vi "CloseIO.vi"   [LabVIEW 2012]
uses:
  <vilib>/Rock Robotics/WPI/RobotDrive/WPI_RobotDriveGetSetRefNum.vi
types:
  T1 = typedef "WPI_UltrasonicDeviceRef.ctl" = cluster{"DevStatus":errorcluster, "Ping Digital Module":T2, "Echo Digital Module":T2, "Ping Channel":T3, "Echo Channel":T3, "CntIndex":T4}
  T2 = typedef "FPGA_TypedefDigitalModule.ctl" = enum16{"Digital Module 1", "Digital Module 2"}
  T3 = typedef "FPGA_DIOChannel.ctl" = enum8{"DIO 1", "DIO 2", "DIO 3", "DIO 4", "DIO 5", "DIO 6", "DIO 7", "DIO 8", "DIO 9", "DIO 10", "DIO 11", "DIO 12", "DIO 13", "DIO 14", "Invalid"}
  T4 = typedef "FPGA_CounterCtrSystemIndex.ctl" = enum8{"Ctr 0", "Ctr 1", "Ctr 2", "Ctr 3", "Ctr 4", "Ctr 5", "Ctr 6", "Ctr 7", "Invalid"}
  T5 = typedef "WPI_MotorControlDeviceRef.ctl" = cluster{"DeviceStatus":errorcluster, "Type":enum16{"PWM", "CAN"}, "PWM":cluster{"Digital Module":T2, "PWM Channel":T6, "DeadBand":T7}, "CAN":cluster{"Device Number":u8, "Control Mode":T8, "Semaphore":T9, "Max Vout":dbl}, "Invert":bool, "TransformRef":T10, "InvTransformRef":T10}
  T6 = typedef "FPGA_DIOPWMChannel.ctl" = enum8{"PWM 1", "PWM 2", "PWM 3", "PWM 4", "PWM 5", "PWM 6", "PWM 7", "PWM 8", "PWM 9", "PWM 10", "Invalid"}
  T7 = typedef "WPI_PWMDeadband.ctl" = cluster{"Name":string, "maxPositivePwm":i32, "minPositivePwm":i32, "centerPwm":i32, "maxNegativePwm":i32, "minNegativePwm":i32, "angularRange":u16}
  T8 = typedef "WPI_CANJaguar_ControlMode.ctl" = enum8{"Percent VBus", "Current", "Speed", "Position", "Voltage"}
  T9 = typedef "Semaphore RefNum" = refnum<k1>
  T10 = typedef "WPI_PWMTransform_ConPane.ctl" = refnum<vi>
  T11 = typedef "WPI_RobotDriveDevRef.ctl" = cluster{"DevStatus":errorcluster, "Motors[]":T5[], "Square Inputs":bool, "Max Output":dbl, "Isochronous":bool}
  T12 = typedef "WPI_DigitalInputDevRef.ctl" = cluster{"DevStatus":errorcluster, "DIO Channel":T3, "Digital Module":T2}
  T13 = typedef "WPI_CounterDevRef.ctl" = cluster{"DevStatus":errorcluster, "CntIndex":T4}
  T14 = typedef "WPI_EncoderDevRef.ctl" = cluster{"DevStatus":errorcluster, "EncoderIndex":T15, "CounterIndex":T4, "DistancePerCount":dbl, "Decoding Type":T16}
  T15 = typedef "FPGA_EncoderIdx.ctl" = enum8{"Enc 0", "Enc 1", "Enc 2", "Enc 3", "Invalid"}
  T16 = typedef "WPI_EncoderType.ctl" = enum16{"1x", "2x", "4x"}
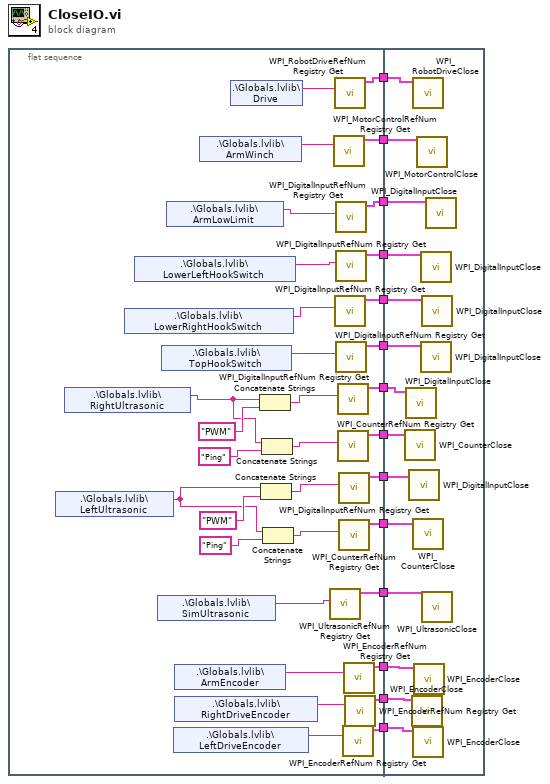
[diagram p0: block diagram]
diagram:
  n1 = flat-sequence {
    tunnel: [w46] -> w14
    tunnel: [w45] -> w13
    tunnel: [w30] -> w12
    tunnel: [w29] -> w11
    tunnel: [w28] -> w10
    tunnel: [w27] -> w9
    tunnel: [w26] -> w8
    tunnel: [w25] -> w7
    tunnel: [w24] -> w6
    tunnel: [w23] -> w5
    tunnel: [w21] -> w4
    tunnel: [w20] -> w3
    tunnel: [w17] -> w2
    tunnel: [w15] -> w1
    tunnel: w14 -> [w62]
    tunnel: w13 -> [w61]
    tunnel: w12 -> [w60]
    tunnel: w11 -> [w59]
    tunnel: w10 -> [w58]
    tunnel: w9 -> [w57]
    tunnel: w8 -> [w56]
    tunnel: w7 -> [w55]
    tunnel: w6 -> [w54]
    tunnel: w5 -> [w53]
    tunnel: w4 -> [w52]
    tunnel: w3 -> [w51]
    tunnel: w2 -> [w50]
    tunnel: w1 -> [w49]
    frame #0 {
      n2 = shared-variable ".\\Globals.lvlib\\LeftUltrasonic"() -> (w32:string)  [unwired: 1 in, 1 out]
      n3 = shared-variable ".\\Globals.lvlib\\RightUltrasonic"() -> (w38:string)  [unwired: 1 in, 1 out]
      n4 = shared-variable ".\\Globals.lvlib\\LowerRightHookSwitch"() -> (w42:string)  [unwired: 1 in, 1 out]
      n5 = shared-variable ".\\Globals.lvlib\\LowerLeftHookSwitch"() -> (w43:string)  [unwired: 1 in, 1 out]
      n6 = shared-variable ".\\Globals.lvlib\\SimUltrasonic"() -> (w16:string)  [unwired: 1 in, 1 out]
      n7 = shared-variable ".\\Globals.lvlib\\TopHookSwitch"() -> (w41:string)  [unwired: 1 in, 1 out]
      n8 = shared-variable ".\\Globals.lvlib\\ArmLowLimit"() -> (w44:string)  [unwired: 1 in, 1 out]
      n9 = shared-variable ".\\Globals.lvlib\\LeftDriveEncoder"() -> (w18:string)  [unwired: 1 in, 1 out]
      n10 = shared-variable ".\\Globals.lvlib\\ArmEncoder"() -> (w19:string)  [unwired: 1 in, 1 out]
      n11 = shared-variable ".\\Globals.lvlib\\RightDriveEncoder"() -> (w22:string)  [unwired: 1 in, 1 out]
      n12 = shared-variable ".\\Globals.lvlib\\ArmWinch"() -> (w47:string)  [unwired: 1 in, 1 out]
      n13 = shared-variable ".\\Globals.lvlib\\Drive"() -> (w48:string)  [unwired: 1 in, 1 out]
      n14 = Concatenate Strings(w38, "PWM") -> (w39:string)
      n15 = Concatenate Strings(w32, "PWM") -> (w34:string)
      n16 = Concatenate Strings(w38, "Ping") -> (w36:string)
      n17 = Concatenate Strings(w32, "Ping") -> (w35:string)
      n18 = call <vilib>:"WPI_UltrasonicRefNum Registry Get.vi"("refnum name"=w16) -> ("UltrasonicDevRef"=w15:T1)  [unwired: 9 in, 1 out]
      n19 = call <vilib>:"WPI_MotorControlRefNum Registry Get.vi"("refnum name"=w47) -> ("MotorControlDevRef"=w45:T5)  [unwired: 9 in, 1 out]
      n20 = call <vilib>:"WPI_RobotDriveRefNum Registry Get.vi"("refnum name"=w48) -> ("RobotDriveDevRef"=w46:T11)  [unwired: 9 in, 1 out]
      n21 = call <vilib>:"WPI_DigitalInputRefNum Registry Get.vi"("refnum name"=w42) -> ("DigitalInputDevRef"=w27:T12)  [unwired: 9 in, 1 out]
      n22 = call <vilib>:"WPI_DigitalInputRefNum Registry Get.vi"("refnum name"=w44) -> ("DigitalInputDevRef"=w25:T12)  [unwired: 9 in, 1 out]
      n23 = call <vilib>:"WPI_DigitalInputRefNum Registry Get.vi"("refnum name"=w43) -> ("DigitalInputDevRef"=w26:T12)  [unwired: 9 in, 1 out]
      n24 = call <vilib>:"WPI_DigitalInputRefNum Registry Get.vi"("refnum name"=w41) -> ("DigitalInputDevRef"=w28:T12)  [unwired: 9 in, 1 out]
      n25 = call <vilib>:"WPI_DigitalInputRefNum Registry Get.vi"("refnum name"=w39) -> ("DigitalInputDevRef"=w29:T12)  [unwired: 9 in, 1 out]
      n26 = call <vilib>:"WPI_CounterRefNum Registry Get.vi"("refnum name"=w36) -> ("CounterDevRef"=w23:T13)  [unwired: 9 in, 1 out]
      n27 = call <vilib>:"WPI_DigitalInputRefNum Registry Get.vi"("refnum name"=w34) -> ("DigitalInputDevRef"=w30:T12)  [unwired: 9 in, 1 out]
      n28 = call <vilib>:"WPI_CounterRefNum Registry Get.vi"("refnum name"=w35) -> ("CounterDevRef"=w24:T13)  [unwired: 9 in, 1 out]
      n29 = call <vilib>:"WPI_EncoderRefNum Registry Get.vi"("refnum name"=w18) -> ("EncoderDevRef"=w17:T14)  [unwired: 9 in, 1 out]
      n30 = call <vilib>:"WPI_EncoderRefNum Registry Get.vi"("refnum name"=w19) -> ("EncoderDevRef"=w20:T14)  [unwired: 9 in, 1 out]
      n31 = call <vilib>:"WPI_EncoderRefNum Registry Get.vi"("refnum name"=w22) -> ("EncoderDevRef"=w21:T14)  [unwired: 9 in, 1 out]
    }
    frame #1 {
      n32 = call <vilib>:"WPI_CounterClose.vi"("CounterDevRef"=w53) -> ()  [unwired: 10 in, 1 out]
      n33 = call <vilib>:"WPI_DigitalInputClose.vi"("DigitalInputDevRef"=w59) -> ()  [unwired: 10 in, 1 out]
      n34 = call <vilib>:"WPI_DigitalInputClose.vi"("DigitalInputDevRef"=w60) -> ()  [unwired: 10 in, 1 out]
      n35 = call <vilib>:"WPI_EncoderClose.vi"("EncoderDevRef"=w52) -> ()  [unwired: 10 in, 1 out]
      n36 = call <vilib>:"WPI_RobotDriveClose.vi"("RobotDriveDevRef"=w62) -> ()  [unwired: 10 in, 1 out]
      n37 = call <vilib>:"WPI_CounterClose.vi"("CounterDevRef"=w54) -> ()  [unwired: 10 in, 1 out]
      n38 = call <vilib>:"WPI_EncoderClose.vi"("EncoderDevRef"=w50) -> ()  [unwired: 10 in, 1 out]
      n39 = call <vilib>:"WPI_EncoderClose.vi"("EncoderDevRef"=w51) -> ()  [unwired: 10 in, 1 out]
      n40 = call <vilib>:"WPI_MotorControlClose.vi"("MotorControlDevRef"=w61) -> ()  [unwired: 10 in, 1 out]
      n41 = call <vilib>:"WPI_DigitalInputClose.vi"("DigitalInputDevRef"=w56) -> ()  [unwired: 10 in, 1 out]
      n42 = call <vilib>:"WPI_DigitalInputClose.vi"("DigitalInputDevRef"=w58) -> ()  [unwired: 10 in, 1 out]
      n43 = call <vilib>:"WPI_DigitalInputClose.vi"("DigitalInputDevRef"=w57) -> ()  [unwired: 10 in, 1 out]
      n44 = call <vilib>:"WPI_UltrasonicClose.vi"("UltrasonicDevRef"=w49) -> ()  [unwired: 10 in, 1 out]
      n45 = call <vilib>:"WPI_DigitalInputClose.vi"("DigitalInputDevRef"=w55) -> ()  [unwired: 10 in, 1 out]
    }
  }
